vi "test sv comm.vi"() -> ()   [LabVIEW 2012]
uses:
  CRDS Class/Main Class/CRDS.lvclass
  CRDS/Controls/CRD State.ctl
panel:
  out "crdClassRef":refnum<data-value>
  out "rt fifo":refnum<k33>
  out "error out":errorcluster
  out "clientTime 2":timestamp
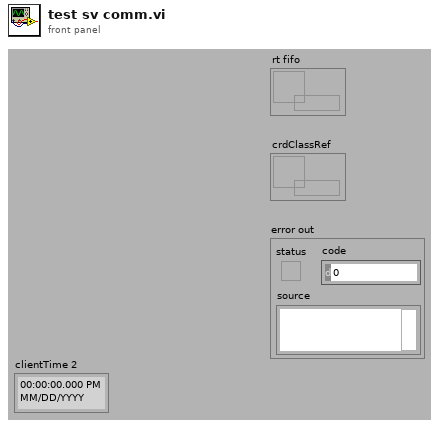
[diagram p1: front panel]
types:
  T1 = enum16{"set date", "set local time", "set UTC time"}
  T2 = typedef "CRD State.ctl" = enum16{"Config", "Init", "Acquire", "Check Time", "Error", "Restart LF AI", "Restart HF AI", "calTau", "calAux", "Update UI", "Write", "Quit"}
  T3 = typedef "LVDateTimeRec.ctl" = cluster{"fractional second":dbl, "second":i32, "minute":i32, "hour":i32, "day of month":i32, "month":i32, "year":i32, "day of week":i32, "day of year":i32, "DST":i32}
  T4 = cluster{"month":i32, "day of month":i32, "year":i32}
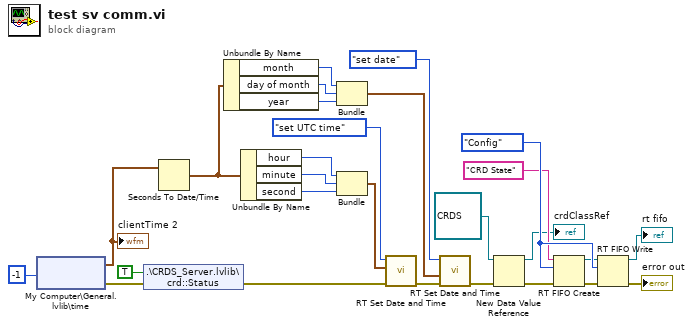
[diagram p0: block diagram]
diagram:
  w18 = CRD_State."Config" ("t")
  n1 = shared-variable "My Computer\\General.lvlib\\time"(-1 ("ms timeout (0)")) -> (w3:timestamp, error out=w2:errorcluster)  [unwired: 1 in, 1 out]
  "clientTime 2" <- w3
  n2 = shared-variable ".\\CRDS_Server.lvlib\\crd::Status"(TRUE ("ServerStart"), error in=w2) -> (error out=w5:errorcluster)
  n3 = Seconds To Date/Time(time stamp (now)=w3) -> (date time rec=w10:T3)  [unwired: 1 in]
  n4 = Unbundle By Name(w10) -> ("month"=w9:i32, "day of month"=w8:i32, "year"=w7:i32)
  n5 = Unbundle By Name(w10) -> ("hour"=w24:i32, "minute"=w25:i32, "second"=w26:i32)
  n6 = Bundle("month"=w9, "day of month"=w8, "year"=w7) -> (w6:T4)  [unwired: 1 in]
  n7 = Bundle("hour"=w24, "minute"=w25, "second"=w26) -> (w23:cluster{"hour":i32, "minute":i32, "second":i32})  [unwired: 1 in]
  n8 = call <vilib>:"RT Set Date and Time.vi"("error in (no error)"=w5, "Time"=w23, "mode"=T1."set UTC time") -> ("error out"=w13:errorcluster)  [unwired: 8 in]
  n9 = call <vilib>:"RT Set Date and Time.vi"("error in (no error)"=w13, "Date"=w6, "mode"=T1."set date") -> ("error out"=w12:errorcluster)  [unwired: 8 in]
  n10 = New Data Value Reference(data value=refnum<class "CRDS.lvclass"> refnum ("CRDS.lvclass"), error in=w12) -> (data value reference=→"crdClassRef":refnum<data-value>, error out=w20:errorcluster)
  n11 = RT FIFO Create(0:"CRD State" ("name (unnamed)"), 1:w18, 3:w20) -> (8:w16:refnum<k33>, 11:w21:errorcluster)  [unwired: 5 in, 1 out]
  n12 = RT FIFO Write(0:w16, 1:w18, 3:w21) -> (8:→"rt fifo":refnum<k33>, 11:→"error out":errorcluster)  [unwired: 2 in, 2 out]
